vi "HackRF_SetBandwith_Filter.vi"(8 "error in (no error)":errorcluster, 10 "FilterBandwidth":dbl format="%#_6p", 11 "HackRF in":T1) -> (0 "error out":errorcluster, 3 "HackRF out":T1)   [LabVIEW 2021]
doc: "Possible values: 1.75/2.5/3.5/5/5.5/6/7/8/9/10/12/14/15/20/24/28MHz,"
uses:
  HackRF_Ref.ctl
  C:/Program Files/HackRF/labview/x64/NetHackrfx64.dll
  NetHackrfx64.dll
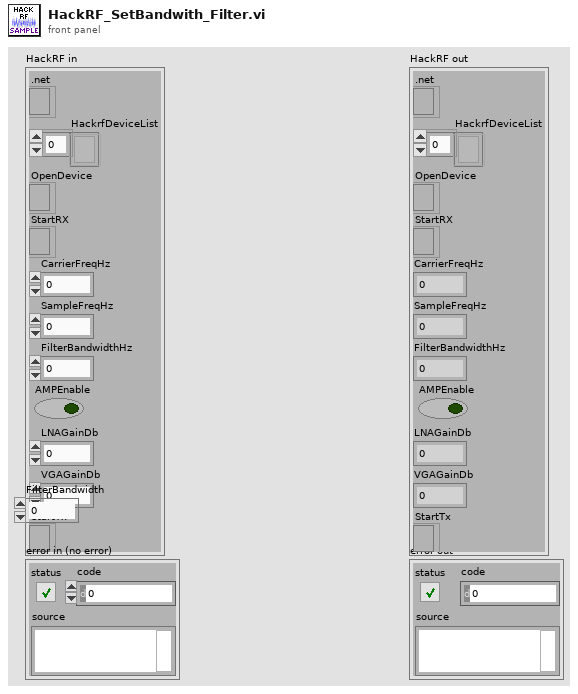
[diagram p1: front panel]
types:
  T1 = typedef "HackRF_Ref.ctl" = cluster{".net":refnum<k24>, "HackrfDeviceList":refnum<k24>[], "OpenDevice":refnum<k24>, "StartRX":refnum<k24>, "CarrierFreqHz":dbl, "SampleFreqHz":dbl, "FilterBandwidthHz":dbl, "AMPEnable":bool, "LNAGainDb":dbl, "VGAGainDb":dbl, "StartTx":refnum<k24>}
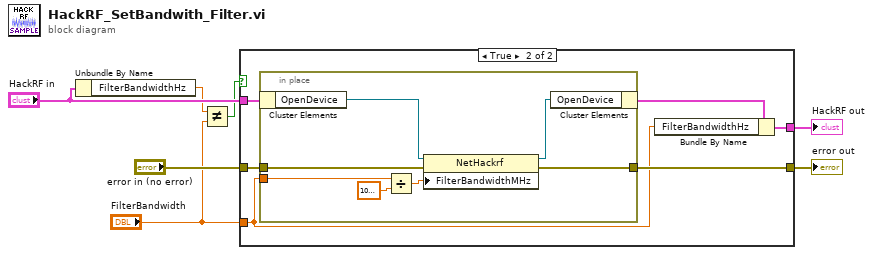
[diagram p0: block diagram]
diagram:
  n1 = Unbundle By Name("HackRF in") -> ("FilterBandwidthHz"=w3:dbl)
  n2 = Not Equal?(x=w3, y="FilterBandwidth") -> (x != y?=w1:bool)
  n3 = case shown="True" w1 {
    tunnel: "error in (no error)" -> [w9 w15]
    tunnel: [w9 w14] -> w6
    tunnel: [w8 w11] -> w5
    tunnel: "HackRF in" -> [w8 w13]
    tunnel: "FilterBandwidth" -> [_ w10]
    frame False {
    }
    frame True {
      n4 = in-place {
        in-place-border: w15 -> [w20]
        in-place-border: [w19] -> w14
        in-place-border: w10 -> [w17]
        n5 = in-place-cluster #1(w13) -> ("OpenDevice"=w22:refnum<k24>)
        n6 = Divide(x=w17, y=1000000.0) -> (x/y=w18:dbl)
        n7 = property class="NetHackrf"(reference=w22, error in=w20, "FilterBandwidthMHz"=w18) -> (reference out=w21:refnum<k24>, error out=w19:errorcluster)
        n8 = in-place-cluster #1("OpenDevice"=w21) -> (w12:T1)
      }
      n9 = Bundle By Name(cluster=w12, "FilterBandwidthHz"=w10) -> (w11:T1)
    }
  }
  "error out" <- w6
  "HackRF out" <- w5
